vi "Set TempSP.vi"(8 "error in (no error)":errorcluster, 10 "Temp SP(C)":dbl, 11 "Modbus Master in":refnum<class "Modbus Master.lvclass">) -> (0 "error out":errorcluster, 3 "Modbus Master out":refnum<class "Modbus Master.lvclass">)   [LabVIEW 2023, in "PIDModbus.lvlib"]
uses:
  PIDModbus.lvlib
  <vilib>/NI/Modbus Library/API/Master/Modbus Master.lvclass
  Controls/Register Enum.ctl
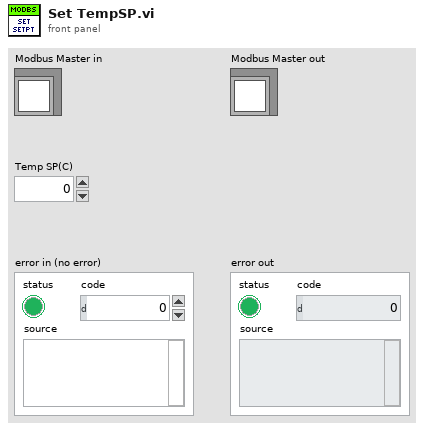
[diagram p1: front panel]
types:
  T1 = typedef "PIDModbus.lvlib/Register Enum.ctl" = u16
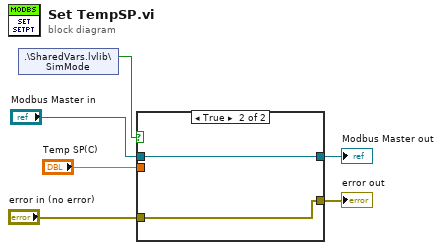
[diagram p0: block diagram]
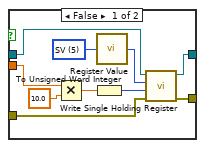
[diagram p2: hidden frame]
diagram:
  n1 = shared-variable ".\\SharedVars.lvlib\\SimMode"() -> (w1:bool)  [unwired: 1 in, 1 out]
  n2 = case shown="True" w1 {
    tunnel: "Temp SP(C)" -> [w13 _]
    tunnel: [w12 w17] -> w5
    tunnel: "error in (no error)" -> [w11 w17]
    tunnel: [w10 w18] -> w3
    tunnel: "Modbus Master in" -> [w9 w18]
    frame False {
      w7 = T1 5 items=["PV"=0, "SV"=5, "P1"=24, "I1"=25, "D1"=26] ("Register")
      n3 = Multiply(x=w13, y=10.0) -> (x*y=w15:dbl)
      n4 = To Unsigned Word Integer(number=w15) -> (unsigned 16bit integer=w16:u16)
      n5 = call "Register Value.vi"("Register"=w7) -> ("RegAddr (Hex)"=w8:u16)
      n6 = call-dynamic "Write Single Holding Register.vi"("error in"=w11, "register to write"=w16, "address"=w8, "Modbus master in"=w9) -> ("error out"=w12:errorcluster, "Modbus master out"=w10:refnum<class "Modbus Master.lvclass">)  [unwired: 6 in]
    }
    frame True {
    }
  }
  "error out" <- w5
  "Modbus Master out" <- w3
